vi "Add Instrument Addon to System Definition File.vi"(8 "error in (no error)":errorcluster, 10 "Instrument Addon Name":string="Instrument Addon", 11 "Instrument Addon Config Datalog Path (.dat)":path) -> (0 "error out":errorcluster, 3 "SysDef Path Out":path)   [LabVIEW 2019, in "Instrument Addon Specific System Tests.lvclass"]
uses:
  Instrument Addon Specific System Tests.lvclass
  APIs/System Definition API/Instrument System Definition API.lvlib
  NationalInstruments.VeriStand.SystemDefinitionAPI
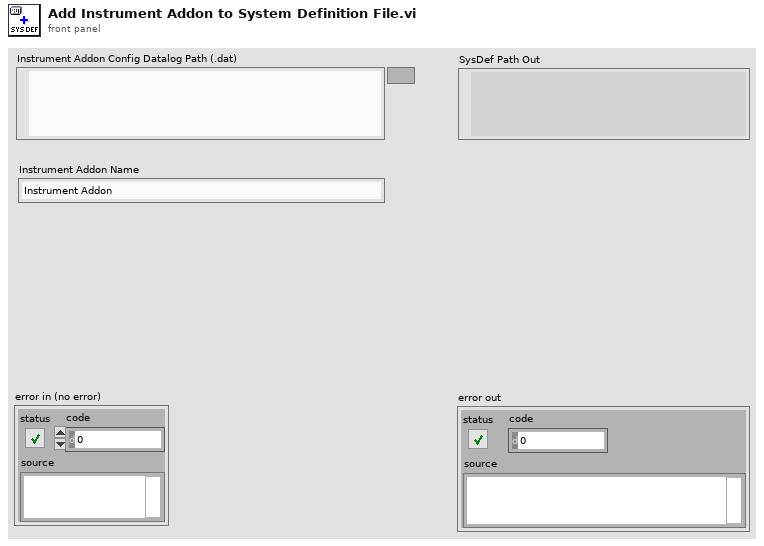
[diagram p1: front panel]
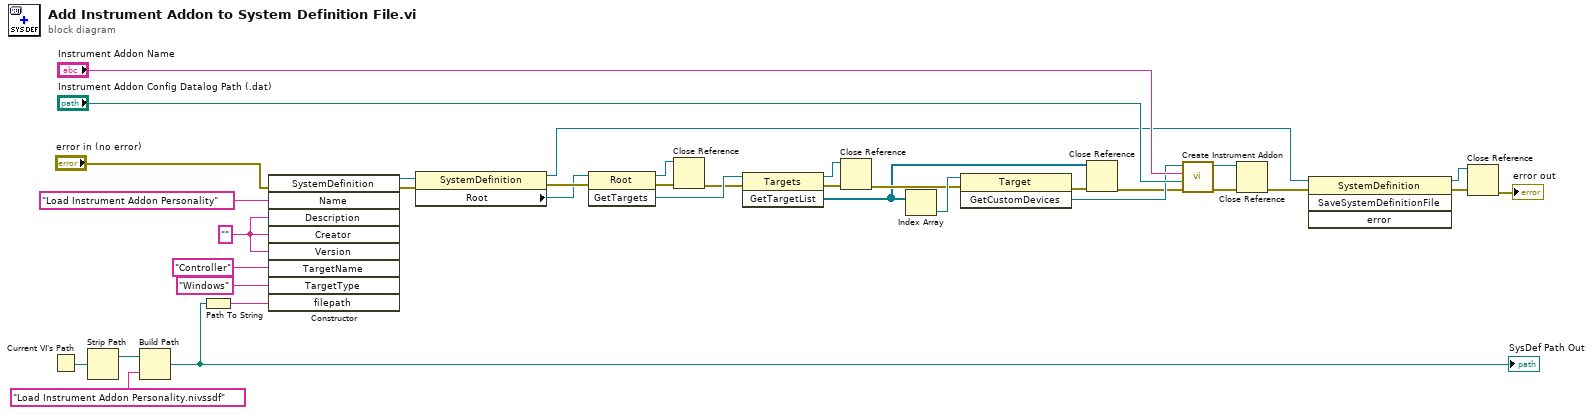
[diagram p0: block diagram]
diagram:
  w6 = "" ("Description")
  n1 = Current VI's Path() -> (path=w11:path)
  n2 = Strip Path(path=w11) -> (stripped path=w10:path)  [unwired: 1 out]
  n3 = Build Path(base path=w10, name or relative path="Load Instrument Addon Personality.nivssdf") -> (appended path=w1:path)
  "SysDef Path Out" <- w1
  n4 = Path To String(path=w1) -> (string=w3:string)
  n5 = constructor class="SystemDefinition"(error in="error in (no error)", "Name"="Load Instrument Addon Personality", "Description"=w6, "Creator"=w6, "Version"=w6, "TargetName"="Controller", "TargetType"="Windows", "filepath"=w3) -> (reference out=w33:refnum<k24>, error out=w32:errorcluster)  [unwired: 2 in, 8 out]
  n6 = property class="SystemDefinition"(reference=w33, error in=w32) -> (reference out=w15:refnum<k24>, error out=w31:errorcluster, "Root"=w8:refnum<k24>)
  n7 = invoke class="Root" method="GetTargets"(reference=w8, error in=w31) -> (reference out=w29:refnum<k24>, error out=w30:errorcluster, "GetTargets"=w28:refnum<k24>)  [unwired: 1 in]
  n8 = Close Reference(reference=w29, error in (no error)=w30) -> (error out=w27:errorcluster)
  n9 = invoke class="Targets" method="GetTargetList"(reference=w28, error in=w27) -> (reference out=w25:refnum<k24>, error out=w26:errorcluster, "GetTargetList"=w22:refnum<k24>[])  [unwired: 1 in]
  n10 = Close Reference(reference=w25, error in (no error)=w26) -> (error out=w23:errorcluster)
  n11 = Index Array(array=w22) -> (element=w24:refnum<k24>)  [unwired: 1 in]
  n12 = invoke class="Target" method="GetCustomDevices"(reference=w24, error in=w23) -> (error out=w21:errorcluster, "GetCustomDevices"=w20:refnum<k24>)  [unwired: 1 in, 1 out]
  n13 = Close Reference(reference=w22, error in (no error)=w21) -> (error out=w19:errorcluster)
  n14 = call "Create Instrument Addon.vi"("error in (no error)"=w19, "CD Config Path (.dat)"="Instrument Addon Config Datalog Path (.dat)", "Name"="Instrument Addon Name", "Custom Devices Ref"=w20) -> ("error out"=w17:errorcluster, "Custom Devices Ref"=w18:refnum<k24>)  [unwired: 6 in]
  n15 = Close Reference(reference=w18, error in (no error)=w17) -> (error out=w16:errorcluster)
  n16 = invoke class="SystemDefinition" method="SaveSystemDefinitionFile"(reference=w15, error in=w16) -> (reference out=w13:refnum<k24>, error out=w14:errorcluster)  [unwired: 2 in, 2 out]
  n17 = Close Reference(reference=w13, error in (no error)=w14) -> (error out=→"error out":errorcluster)
